vi "Eurotherm_2023_Module.vi"(4 "Decimales":u16(ring)=1 items=["0"=1, "1"=10, "2"=100], 5 "Eurotherm (T:Enable)":bool=TRUE, 6 "delay(s)":dbl=0.15 format="%#_13g", 7 "Command":T3, 8 "error in (no error)":errorcluster, 9 "Value":dbl format="%04.1g", 10 "Address":T1, 11 "VISA resource name":refnum<visa-resource-name>) -> (0 "error out":errorcluster, 2 "Eurotherm":T2, 3 "Valid":bool)   [LabVIEW 2017]
uses:
  Eurotherm_2023_Module.ctl
  Address.ctl
  <vilib>/Instr/_visa.llb/VISA Configure Serial Port (Instr).vi
panel:
  out "String Read":string
  out "String Write":string
  # "NUEVO MODULO VI\nQUE INCORPORA LÍMITES DE SALIDA"
  # "Eurotherm New Module"
  # "Input Data"
  # "Local Data"
  # "Output Data"
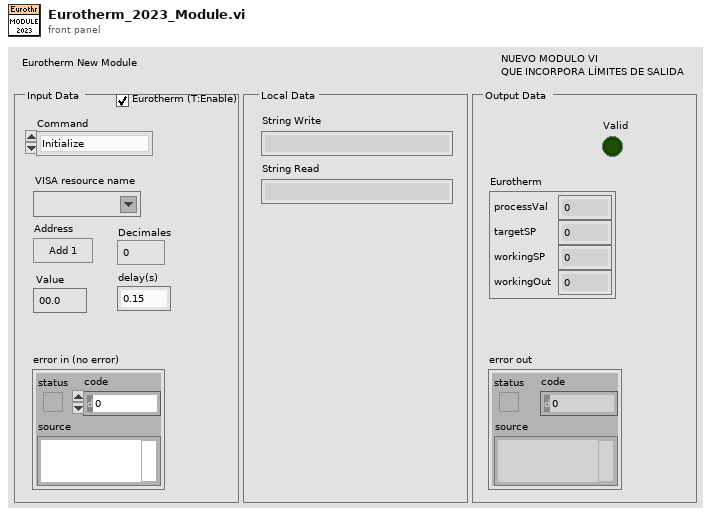
[diagram p1: front panel]
types:
  T1 = typedef "Address.ctl" = enum16{"Add 1", "Add 2", "Add 3", "Add 4", "Add 5", "Add 6", "Add 10", "Add 11", "Add 12", "Add 13"}
  T2 = cluster{"processVal":dbl, "targetSP":dbl, "workingSP":dbl, "workingOut":dbl}
  T3 = typedef "Eurotherm_2023_Module.ctl" = enum16{"Initialize", "Write setpoint", "Read data", "Write ramp rate", "Set constante proporcional", "Set constante integral", "Set constante diferencial", "Set ouput limit LOW", "Set ouput limit HIGH", "Shutdown"}
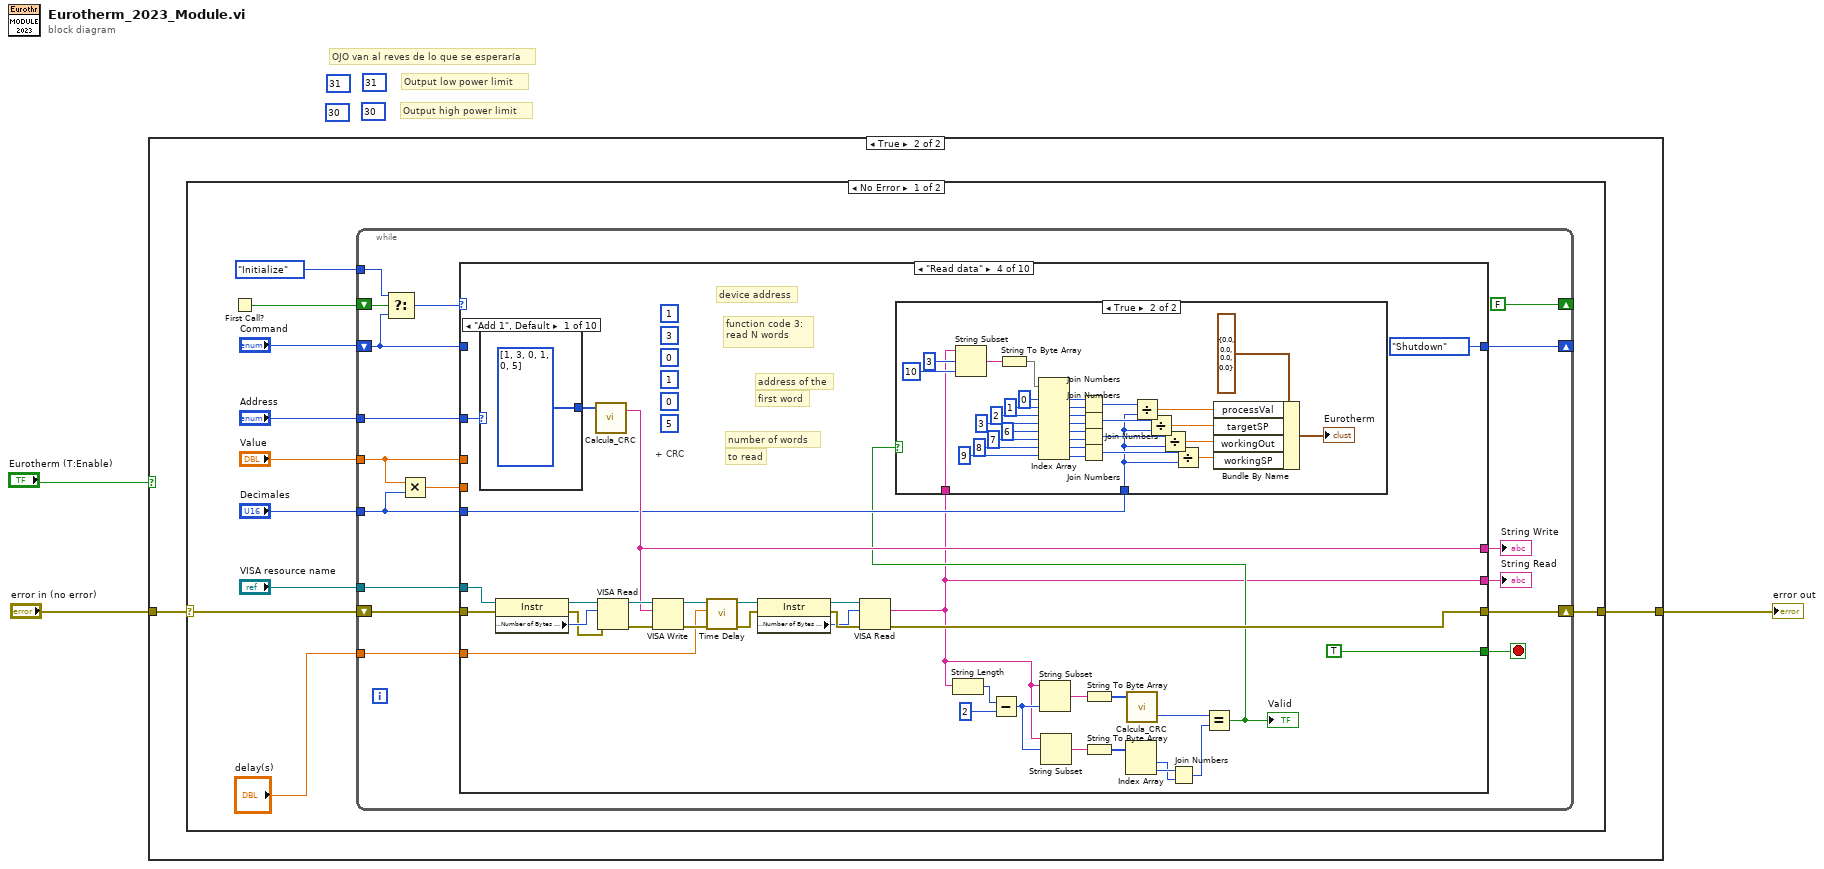
[diagram p0: block diagram]
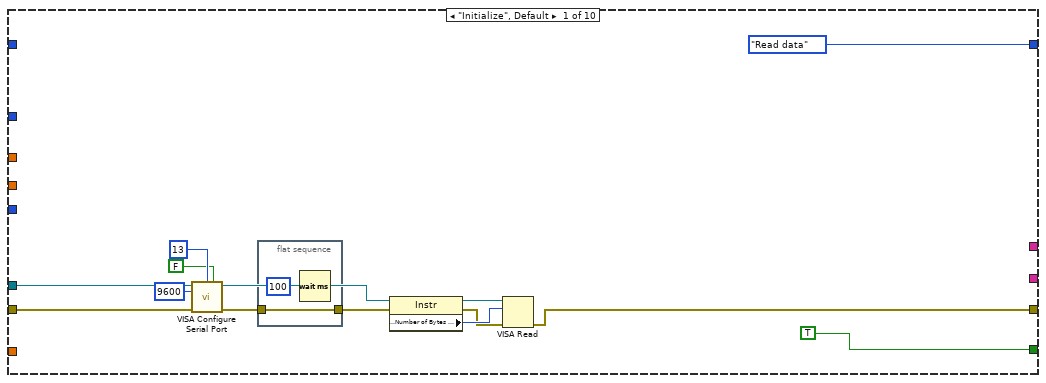
[diagram p3: hidden frame]
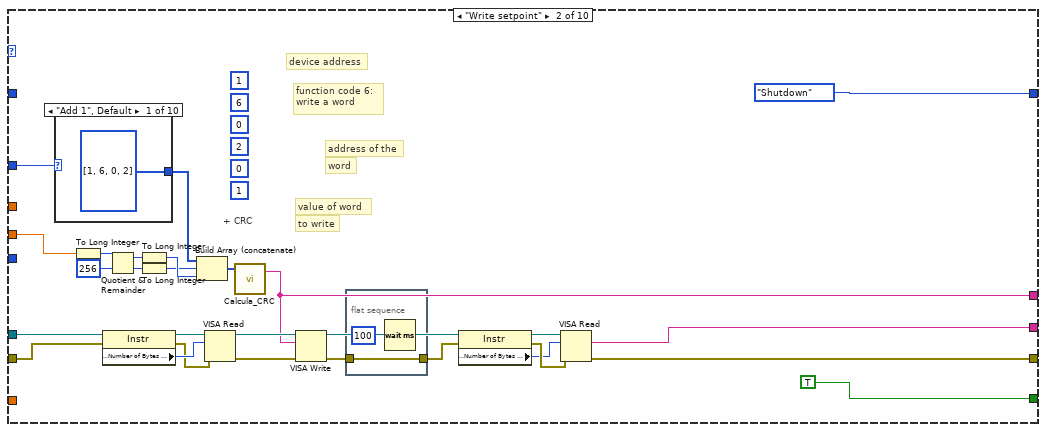
[diagram p4: hidden frame]
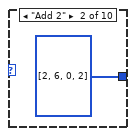
[diagram p5: hidden frame]
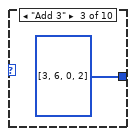
[diagram p6: hidden frame]
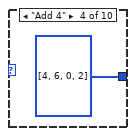
[diagram p7: hidden frame]
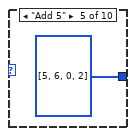
[diagram p8: hidden frame]
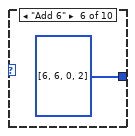
[diagram p9: hidden frame]
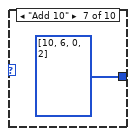
[diagram p10: hidden frame]
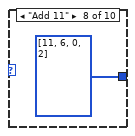
[diagram p11: hidden frame]
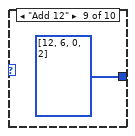
[diagram p12: hidden frame]
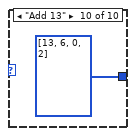
[diagram p13: hidden frame]
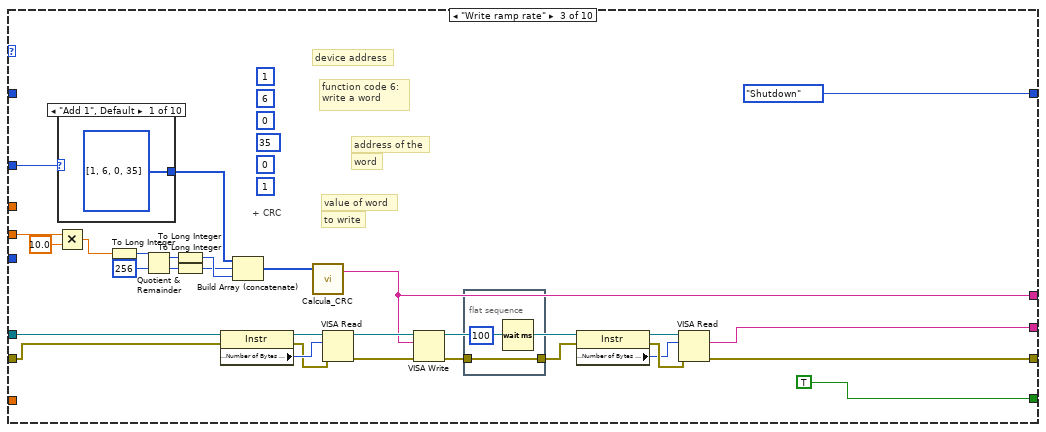
[diagram p14: hidden frame]
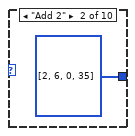
[diagram p15: hidden frame]
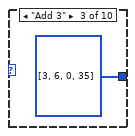
[diagram p16: hidden frame]
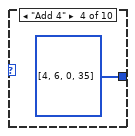
[diagram p17: hidden frame]
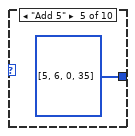
[diagram p18: hidden frame]
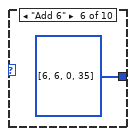
[diagram p19: hidden frame]
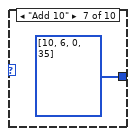
[diagram p20: hidden frame]
diagram:
  (unwired) u8 30
  (unwired) u8 31
  (unwired) u8 30
  (unwired) u8 31
  # "OJO van al reves de lo que se esperaría"
  # "Output high power limit"
  # "Output low power limit"
  n1 = case shown="True" "Eurotherm (T:Enable)" {
    tunnel: "error in (no error)" -> [w4 w6]
    tunnel: [w4 w5] -> w2
    frame False {
    }
    frame True {
      n2 = case shown="No Error" w6 {
        selector: w6 -> [w15 w413]
        tunnel: [w14 w413] -> w5
        frame No Error {
          n3 = First Call?() -> (First Call?: T/F=w16:bool)
          n4 = while {
            shift-right: [w28] -> _
            shift-left: "Command" -> [w29]
            shift-right: [w26] -> w14
            shift-left: w15 -> [w25]
            shift-right: [FALSE ("First Call?: T/F")] -> _
            shift-left: w16 -> [w33]
            tunnel: Eurotherm_2023_Module."Initialize" ("Command") -> [w32]
            tunnel: "Address" -> [w22]
            tunnel: "Value" -> [w19]
            tunnel: "Decimales" -> [w21]
            tunnel: "VISA resource name" -> [w18]
            tunnel: "delay(s)" -> [w17]
            stop <- w27 stop-if-true
            n5 = Select(t=w32, s=w33, f=w29) -> (s? t:f=w30:T3)
            n6 = Multiply(x=w19, y=w21) -> (x*y=w20:dbl)
            n7 = case shown="\"Read data\"" w30 {
              tunnel: w29 -> [_ _ _ _ _ _ _ _ _ _]
              tunnel: [Eurotherm_2023_Module."Read data" ("Command") Eurotherm_2023_Module."Shutdown" ("Command") Eurotherm_2023_Module."Shutdown" ("Command") Eurotherm_2023_Module."Shutdown" ("Command") Eurotherm_2023_Module."Shutdown" ("Command") Eurotherm_2023_Module."Shutdown" ("Command") Eurotherm_2023_Module."Shutdown" ("Command") Eurotherm_2023_Module."Shutdown" ("Command") Eurotherm_2023_Module."Shutdown" ("Command") Eurotherm_2023_Module."Shutdown" ("Command")] -> w28
              tunnel: [TRUE ("First Call?: T/F") TRUE ("First Call?: T/F") TRUE ("First Call?: T/F") TRUE ("First Call?: T/F") TRUE ("First Call?: T/F") TRUE ("First Call?: T/F") TRUE ("First Call?: T/F") TRUE ("First Call?: T/F") TRUE ("First Call?: T/F") TRUE ("First Call?: T/F")] -> w27
              tunnel: [w37 w57 w96 w150 w215 w255 w295 w335 w375 w409] -> w26
              tunnel: w25 -> [w38 w58 w99 w154 w216 w256 w296 w336 w376 w410]
              tunnel: w18 -> [w35 w56 w100 w153 w214 w254 w294 w334 w374 w411]
              tunnel: [_ w55 w95 w132 w213 w253 w293 w333 w373 _] -> w24
              tunnel: [_ w54 w94 w152 w212 w252 w292 w332 w372 _] -> w23
              tunnel: w22 -> [_ w52 w98 w165 w210 w250 w290 w330 w370 _]
              tunnel: w20 -> [_ w51 w93 _ _ _ _ _ _ _]
              tunnel: w21 -> [_ _ _ w146 _ _ _ _ _ _]
              tunnel: w19 -> [_ _ _ _ w209 w249 w289 w329 w369 _]
              tunnel: w17 -> [_ _ _ w147 _ _ _ _ _ _]
              frame "Initialize", Default {
                n8 = call-poly "VISA Configure Serial Port"("VISA resource name"=w35, "termination char\n(0xA = '\\n' = LF)"=u8 13 ("termination char\n(0xA = '\\n' = LF)"), "Enable Termination\nChar (T)"=FALSE ("Enable Termination\nChar (T)"), "baud rate (9600)"=u32 9600, "error in (no error)"=w38) -> ("VISA resource name out"=w39:refnum<visa-resource-name>, "error out"=w40:errorcluster)  [unwired: 9 in]
                n9 = flat-sequence {
                  tunnel: w40 -> [w48]
                  tunnel: [w48] -> w47
                  frame #0 {
                    n10 = Wait (ms)(milliseconds to wait=u32 100) -> ()  [unwired: 1 out]
                  }
                }
                n11 = property class="Instr"(reference=w39, error in=w47) -> (reference out=w44:refnum<visa-resource-name>, error out=w45:errorcluster, "Serial Settings:Number of Bytes at Serial Port"=w46:u32)
                n12 = VISA Read(VISA resource name=w44, byte count=w46, error in (no error)=w45) -> (error out=w37:errorcluster)  [unwired: 3 out]
              }
              frame "Write setpoint" {
                (unwired) 1
                (unwired) u8 0
                (unwired) 2
                (unwired) u8 0
                (unwired) 6
                (unwired) u8 1
                # "+ CRC"
                # "to write"
                # "value of word"
                # "word"
                # "address of the"
                # "function code 6:\nwrite a word"
                # "device address"
                n13 = case shown="\"Add 1\", Default" w52 {
                  tunnel: [u8[] [1, 6, 0, 2] ("Message Data") u8[] [2, 6, 0, 2] ("Message Data") u8[] [3, 6, 0, 2] ("Message Data") u8[] [4, 6, 0, 2] ("Message Data") u8[] [5, 6, 0, 2] ("Message Data") u8[] [6, 6, 0, 2] ("Message Data") u8[] [10, 6, 0, 2] ("Message Data") u8[] [11, 6, 0, 2] ("Message Data") u8[] [12, 6, 0, 2] ("Message Data") u8[] [13, 6, 0, 2] ("Message Data")] -> w77
                  frame "Add 1", Default {
                  }
                  frame "Add 2" {
                  }
                  frame "Add 3" {
                  }
                  frame "Add 4" {
                  }
                  frame "Add 5" {
                  }
                  frame "Add 6" {
                  }
                  frame "Add 10" {
                  }
                  frame "Add 11" {
                  }
                  frame "Add 12" {
                  }
                  frame "Add 13" {
                  }
                }
                n14 = To Long Integer(number=w51) -> (32bit integer=w76:i32)
                n15 = property class="Instr"(reference=w56, error in=w58) -> (reference out=w59:refnum<visa-resource-name>, error out=w60:errorcluster, "Serial Settings:Number of Bytes at Serial Port"=w61:u32)
                n16 = Quotient & Remainder(x=w76, y=256) -> (x-y*floor(x/y)=w71:i32, floor(x/y)=w72:i32)
                n17 = To Long Integer(number=w71) -> (32bit integer=w74:i32)
                n18 = To Long Integer(number=w72) -> (32bit integer=w73:i32)
                n19 = Build Array (concatenate)(w77, w73, w74) -> (w75:i32[])
                n20 = VISA Read(VISA resource name=w59, byte count=w61, error in (no error)=w60) -> (VISA resource name out=w68:refnum<visa-resource-name>, error out=w67:errorcluster)  [unwired: 2 out]
                n21 = call "Calcula_CRC.vi"("Message Data"=w75) -> ("String"=w54:string)  [unwired: 2 in, 1 out]
                n22 = VISA Write(VISA resource name=w68, write buffer=w54, error in (no error)=w67) -> (VISA resource name out=w69:refnum<visa-resource-name>, error out=w66:errorcluster)  [unwired: 1 out]
                n23 = flat-sequence {
                  tunnel: w66 -> [w78]
                  tunnel: [w78] -> w65
                  frame #0 {
                    n24 = Wait (ms)(milliseconds to wait=u32 100) -> ()  [unwired: 1 out]
                  }
                }
                n25 = property class="Instr"(reference=w69, error in=w65) -> (reference out=w64:refnum<visa-resource-name>, error out=w63:errorcluster, "Serial Settings:Number of Bytes at Serial Port"=w62:u32)
                n26 = VISA Read(VISA resource name=w64, byte count=w62, error in (no error)=w63) -> (read buffer=w55:string, error out=w57:errorcluster)  [unwired: 2 out]
              }
              frame "Write ramp rate" {
                (unwired) 1
                (unwired) u8 0
                (unwired) 35
                (unwired) u8 0
                (unwired) 6
                (unwired) u8 1
                # "+ CRC"
                # "to write"
                # "value of word"
                # "word"
                # "address of the"
                # "function code 6:\nwrite a word"
                # "device address"
                n27 = Multiply(x=w93, y=10.0) -> (x*y=w92:dbl)
                n28 = case shown="\"Add 1\", Default" w98 {
                  tunnel: [u8[] [1, 6, 0, 35] ("Message Data") u8[] [2, 6, 0, 35] ("Message Data") u8[] [3, 6, 0, 35] ("Message Data") u8[] [4, 6, 0, 35] ("Message Data") u8[] [5, 6, 0, 35] ("Message Data") u8[] [6, 6, 0, 35] ("Message Data") u8[] [10, 6, 0, 35] ("Message Data") u8[] [11, 6, 0, 35] ("Message Data") u8[] [12, 6, 0, 35] ("Message Data") u8[] [13, 6, 0, 35] ("Message Data")] -> w119
                  frame "Add 1", Default {
                  }
                  frame "Add 2" {
                  }
                  frame "Add 3" {
                  }
                  frame "Add 4" {
                  }
                  frame "Add 5" {
                  }
                  frame "Add 6" {
                  }
                  frame "Add 10" {
                  }
                  frame "Add 11" {
                  }
                  frame "Add 12" {
                  }
                  frame "Add 13" {
                  }
                }
                n29 = To Long Integer(number=w92) -> (32bit integer=w118:i32)
                n30 = Quotient & Remainder(x=w118, y=256) -> (x-y*floor(x/y)=w113:i32, floor(x/y)=w114:i32)
                n31 = To Long Integer(number=w113) -> (32bit integer=w116:i32)
                n32 = To Long Integer(number=w114) -> (32bit integer=w115:i32)
                n33 = property class="Instr"(reference=w100, error in=w99) -> (reference out=w101:refnum<visa-resource-name>, error out=w102:errorcluster, "Serial Settings:Number of Bytes at Serial Port"=w103:u32)
                n34 = Build Array (concatenate)(w119, w115, w116) -> (w117:i32[])
                n35 = call "Calcula_CRC.vi"("Message Data"=w117) -> ("String"=w94:string)  [unwired: 2 in, 1 out]
                n36 = VISA Read(VISA resource name=w101, byte count=w103, error in (no error)=w102) -> (VISA resource name out=w110:refnum<visa-resource-name>, error out=w109:errorcluster)  [unwired: 2 out]
                n37 = VISA Write(VISA resource name=w110, write buffer=w94, error in (no error)=w109) -> (VISA resource name out=w111:refnum<visa-resource-name>, error out=w108:errorcluster)  [unwired: 1 out]
                n38 = flat-sequence {
                  tunnel: w108 -> [w120]
                  tunnel: [w120] -> w107
                  frame #0 {
                    n39 = Wait (ms)(milliseconds to wait=u32 100) -> ()  [unwired: 1 out]
                  }
                }
                n40 = property class="Instr"(reference=w111, error in=w107) -> (reference out=w106:refnum<visa-resource-name>, error out=w105:errorcluster, "Serial Settings:Number of Bytes at Serial Port"=w104:u32)
                n41 = VISA Read(VISA resource name=w106, byte count=w104, error in (no error)=w105) -> (read buffer=w95:string, error out=w96:errorcluster)  [unwired: 2 out]
              }
              frame "Read data" {
                (unwired) u8 5
                (unwired) u8 0
                (unwired) u8 1
                (unwired) u8 0
                (unwired) u8 3
                (unwired) u8 1
                # "+ CRC"
                # "to read"
                # "number of words"
                # "first word"
                # "address of the"
                # "function code 3:\nread N words"
                # "device address"
                n42 = case shown="\"Add 1\", Default" w165 {
                  tunnel: [u8[] [1, 3, 0, 1, 0, 5] ("Message Data") u8[] [2, 3, 0, 1, 0, 5] ("Message Data") u8[] [3, 3, 0, 1, 0, 5] ("Message Data") u8[] [4, 3, 0, 1, 0, 5] ("Message Data") u8[] [5, 3, 0, 1, 0, 5] ("Message Data") u8[] [6, 3, 0, 1, 0, 5] ("Message Data") u8[] [10, 3, 0, 1, 0, 5] ("Message Data") u8[] [11, 3, 0, 1, 0, 5] ("Message Data") u8[] [12, 3, 0, 1, 0, 5] ("Message Data") u8[] [13, 3, 0, 1, 0, 5] ("Message Data")] -> w164
                  frame "Add 1", Default {
                  }
                  frame "Add 2" {
                  }
                  frame "Add 3" {
                  }
                  frame "Add 4" {
                  }
                  frame "Add 5" {
                  }
                  frame "Add 6" {
                  }
                  frame "Add 10" {
                  }
                  frame "Add 11" {
                  }
                  frame "Add 12" {
                  }
                  frame "Add 13" {
                  }
                }
                n43 = property class="Instr"(reference=w153, error in=w154) -> (reference out=w155:refnum<visa-resource-name>, error out=w156:errorcluster, "Serial Settings:Number of Bytes at Serial Port"=w157:u32)
                n44 = call "Calcula_CRC.vi"("Message Data"=w164) -> ("String"=w152:string)  [unwired: 2 in, 1 out]
                n45 = VISA Read(VISA resource name=w155, byte count=w157, error in (no error)=w156) -> (VISA resource name out=w162:refnum<visa-resource-name>, error out=w161:errorcluster)  [unwired: 2 out]
                n46 = VISA Write(VISA resource name=w162, write buffer=w152, error in (no error)=w161) -> (VISA resource name out=w163:refnum<visa-resource-name>, error out=w149:errorcluster)  [unwired: 1 out]
                n47 = call "Time Delay"("error in (no error)"=w149, "Delay Time (s)"=w147) -> ("error out"=w148:errorcluster)  [unwired: 9 in]
                n48 = property class="Instr"(reference=w163, error in=w148) -> (reference out=w160:refnum<visa-resource-name>, error out=w159:errorcluster, "Serial Settings:Number of Bytes at Serial Port"=w158:u32)
                n49 = VISA Read(VISA resource name=w160, byte count=w158, error in (no error)=w159) -> (read buffer=w132:string, error out=w150:errorcluster)  [unwired: 2 out]
                n50 = String Length(string=w132) -> (length=w144:i32)
                n51 = Subtract(x=w144, y=2) -> (x-y=w143:i32)
                n52 = String Subset(string=w132, length (rest)=w143) -> (substring=w142:string)  [unwired: 1 in]
                n53 = String Subset(string=w132, offset (0)=w143) -> (substring=w140:string)  [unwired: 1 in]
                n54 = String To Byte Array(string=w142) -> (unsigned byte array=w141:u8[])
                n55 = String To Byte Array(string=w140) -> (unsigned byte array=w139:u8[])
                n56 = Index Array(array=w139) -> (element #1=w137:u8, element #2=w138:u8)  [unwired: 2 in]
                n57 = call "Calcula_CRC.vi"("Message Data"=w141) -> ("Calculated CRC"=w136:u16)  [unwired: 2 in, 1 out]
                n58 = Join Numbers(hi=w138, lo=w137) -> ((hi.lo)=w135:u16)
                n59 = Equal?(x=w136, y=w135) -> (x = y?=w133:bool)
                "Valid" <- w133
                n60 = case shown="True" w133 {
                  tunnel: w132 -> [_ w191]
                  tunnel: w146 -> [_ w172]
                  frame False {
                  }
                  frame True {
                    n61 = String Subset(string=w191, offset (0)=3, length (rest)=10 ("length (rest)")) -> (substring=w192:string)
                    n62 = String To Byte Array(string=w192) -> (unsigned byte array=w195:u8[])
                    n63 = Index Array(array=w195, index #1=0 ("index"), index #2=1 ("index"), index #3=2 ("index"), index #4=3 ("index"), index #5=6 ("index"), index #6=7 ("index"), index #7=8 ("index"), index #8=9 ("index")) -> (element #1=w184:u8, element #2=w183:u8, element #3=w182:u8, element #4=w181:u8, element #5=w180:u8, element #6=w179:u8, element #7=w178:u8, element #8=w177:u8)
                    n64 = Join Numbers(hi=w184, lo=w183) -> ((hi.lo)=w176:u16)
                    n65 = Join Numbers(hi=w182, lo=w181) -> ((hi.lo)=w175:u16)
                    n66 = Join Numbers(hi=w180, lo=w179) -> ((hi.lo)=w174:u16)
                    n67 = Join Numbers(hi=w178, lo=w177) -> ((hi.lo)=w173:u16)
                    n68 = Divide(x=w176, y=w172) -> (x/y=w166:dbl)
                    n69 = Divide(x=w175, y=w172) -> (x/y=w167:dbl)
                    n70 = Divide(x=w174, y=w172) -> (x/y=w168:dbl)
                    n71 = Divide(x=w173, y=w172) -> (x/y=w169:dbl)
                    n72 = Bundle By Name(cluster=T2 {"processVal"=0.0, "targetSP"=0.0, "workingSP"=0.0, "workingOut"=0.0} ("Eurotherm"), "processVal"=w166, "targetSP"=w167, "workingOut"=w168, "workingSP"=w169) -> (→"Eurotherm":T2)
                  }
                }
              }
              frame "Set constante proporcional" {
                (unwired) 1
                (unwired) u8 0
                (unwired) 6
                (unwired) u8 0
                (unwired) 6
                (unwired) u8 1
                # "+ CRC"
                # "to write"
                # "value of word"
                # "word"
                # "address of the"
                # "function code 6:\nwrite a word"
                # "device address"
                n73 = case shown="\"Add 1\", Default" w210 {
                  tunnel: [u8[] [1, 6, 0, 6] ("Message Data") u8[] [2, 6, 0, 6] ("Message Data") u8[] [3, 6, 0, 6] ("Message Data") u8[] [4, 6, 0, 6] ("Message Data") u8[] [5, 6, 0, 6] ("Message Data") u8[] [6, 6, 0, 6] ("Message Data") u8[] [10, 6, 0, 6] ("Message Data") u8[] [11, 6, 0, 6] ("Message Data") u8[] [12, 6, 0, 6] ("Message Data") u8[] [13, 6, 0, 6] ("Message Data")] -> w235
                  frame "Add 1", Default {
                  }
                  frame "Add 2" {
                  }
                  frame "Add 3" {
                  }
                  frame "Add 4" {
                  }
                  frame "Add 5" {
                  }
                  frame "Add 6" {
                  }
                  frame "Add 10" {
                  }
                  frame "Add 11" {
                  }
                  frame "Add 12" {
                  }
                  frame "Add 13" {
                  }
                }
                n74 = To Long Integer(number=w209) -> (32bit integer=w234:i32)
                n75 = property class="Instr"(reference=w214, error in=w216) -> (reference out=w217:refnum<visa-resource-name>, error out=w218:errorcluster, "Serial Settings:Number of Bytes at Serial Port"=w219:u32)
                n76 = Quotient & Remainder(x=w234, y=256) -> (x-y*floor(x/y)=w229:i32, floor(x/y)=w230:i32)
                n77 = To Long Integer(number=w229) -> (32bit integer=w232:i32)
                n78 = To Long Integer(number=w230) -> (32bit integer=w231:i32)
                n79 = Build Array (concatenate)(w235, w231, w232) -> (w233:i32[])
                n80 = VISA Read(VISA resource name=w217, byte count=w219, error in (no error)=w218) -> (VISA resource name out=w226:refnum<visa-resource-name>, error out=w225:errorcluster)  [unwired: 2 out]
                n81 = call "Calcula_CRC.vi"("Message Data"=w233) -> ("String"=w212:string)  [unwired: 2 in, 1 out]
                n82 = VISA Write(VISA resource name=w226, write buffer=w212, error in (no error)=w225) -> (VISA resource name out=w227:refnum<visa-resource-name>, error out=w224:errorcluster)  [unwired: 1 out]
                n83 = flat-sequence {
                  tunnel: w224 -> [w236]
                  tunnel: [w236] -> w223
                  frame #0 {
                    n84 = Wait (ms)(milliseconds to wait=u32 100) -> ()  [unwired: 1 out]
                  }
                }
                n85 = property class="Instr"(reference=w227, error in=w223) -> (reference out=w222:refnum<visa-resource-name>, error out=w221:errorcluster, "Serial Settings:Number of Bytes at Serial Port"=w220:u32)
                n86 = VISA Read(VISA resource name=w222, byte count=w220, error in (no error)=w221) -> (read buffer=w213:string, error out=w215:errorcluster)  [unwired: 2 out]
              }
              frame "Set constante integral" {
                (unwired) 1
                (unwired) u8 0
                (unwired) 8
                (unwired) u8 0
                (unwired) 6
                (unwired) u8 1
                # "+ CRC"
                # "to write"
                # "value of word"
                # "word"
                # "address of the"
                # "function code 6:\nwrite a word"
                # "device address"
                n87 = case shown="\"Add 1\", Default" w250 {
                  tunnel: [u8[] [1, 6, 0, 8] ("Message Data") u8[] [2, 6, 0, 8] ("Message Data") u8[] [3, 6, 0, 8] ("Message Data") u8[] [4, 6, 0, 8] ("Message Data") u8[] [5, 6, 0, 8] ("Message Data") u8[] [6, 6, 0, 8] ("Message Data") u8[] [10, 6, 0, 8] ("Message Data") u8[] [11, 6, 0, 8] ("Message Data") u8[] [12, 6, 0, 8] ("Message Data") u8[] [13, 6, 0, 8] ("Message Data")] -> w275
                  frame "Add 1", Default {
                  }
                  frame "Add 2" {
                  }
                  frame "Add 3" {
                  }
                  frame "Add 4" {
                  }
                  frame "Add 5" {
                  }
                  frame "Add 6" {
                  }
                  frame "Add 10" {
                  }
                  frame "Add 11" {
                  }
                  frame "Add 12" {
                  }
                  frame "Add 13" {
                  }
                }
                n88 = To Long Integer(number=w249) -> (32bit integer=w274:i32)
                n89 = property class="Instr"(reference=w254, error in=w256) -> (reference out=w257:refnum<visa-resource-name>, error out=w258:errorcluster, "Serial Settings:Number of Bytes at Serial Port"=w259:u32)
                n90 = Quotient & Remainder(x=w274, y=256) -> (x-y*floor(x/y)=w269:i32, floor(x/y)=w270:i32)
                n91 = To Long Integer(number=w269) -> (32bit integer=w272:i32)
                n92 = To Long Integer(number=w270) -> (32bit integer=w271:i32)
                n93 = Build Array (concatenate)(w275, w271, w272) -> (w273:i32[])
                n94 = VISA Read(VISA resource name=w257, byte count=w259, error in (no error)=w258) -> (VISA resource name out=w266:refnum<visa-resource-name>, error out=w265:errorcluster)  [unwired: 2 out]
                n95 = call "Calcula_CRC.vi"("Message Data"=w273) -> ("String"=w252:string)  [unwired: 2 in, 1 out]
                n96 = VISA Write(VISA resource name=w266, write buffer=w252, error in (no error)=w265) -> (VISA resource name out=w267:refnum<visa-resource-name>, error out=w264:errorcluster)  [unwired: 1 out]
                n97 = flat-sequence {
                  tunnel: w264 -> [w276]
                  tunnel: [w276] -> w263
                  frame #0 {
                    n98 = Wait (ms)(milliseconds to wait=u32 100) -> ()  [unwired: 1 out]
                  }
                }
                n99 = property class="Instr"(reference=w267, error in=w263) -> (reference out=w262:refnum<visa-resource-name>, error out=w261:errorcluster, "Serial Settings:Number of Bytes at Serial Port"=w260:u32)
                n100 = VISA Read(VISA resource name=w262, byte count=w260, error in (no error)=w261) -> (read buffer=w253:string, error out=w255:errorcluster)  [unwired: 2 out]
              }
              frame "Set constante diferencial" {
                (unwired) 1
                (unwired) u8 0
                (unwired) 9
                (unwired) u8 0
                (unwired) 6
                (unwired) u8 1
                # "+ CRC"
                # "to write"
                # "value of word"
                # "word"
                # "address of the"
                # "function code 6:\nwrite a word"
                # "device address"
                n101 = case shown="\"Add 1\", Default" w290 {
                  tunnel: [u8[] [1, 6, 0, 9] ("Message Data") u8[] [2, 6, 0, 9] ("Message Data") u8[] [3, 6, 0, 9] ("Message Data") u8[] [4, 6, 0, 9] ("Message Data") u8[] [5, 6, 0, 9] ("Message Data") u8[] [6, 6, 0, 9] ("Message Data") u8[] [10, 6, 0, 9] ("Message Data") u8[] [11, 6, 0, 9] ("Message Data") u8[] [12, 6, 0, 9] ("Message Data") u8[] [13, 6, 0, 9] ("Message Data")] -> w315
                  frame "Add 1", Default {
                  }
                  frame "Add 2" {
                  }
                  frame "Add 3" {
                  }
                  frame "Add 4" {
                  }
                  frame "Add 5" {
                  }
                  frame "Add 6" {
                  }
                  frame "Add 10" {
                  }
                  frame "Add 11" {
                  }
                  frame "Add 12" {
                  }
                  frame "Add 13" {
                  }
                }
                n102 = To Long Integer(number=w289) -> (32bit integer=w314:i32)
                n103 = property class="Instr"(reference=w294, error in=w296) -> (reference out=w297:refnum<visa-resource-name>, error out=w298:errorcluster, "Serial Settings:Number of Bytes at Serial Port"=w299:u32)
                n104 = Quotient & Remainder(x=w314, y=256) -> (x-y*floor(x/y)=w309:i32, floor(x/y)=w310:i32)
                n105 = To Long Integer(number=w309) -> (32bit integer=w312:i32)
                n106 = To Long Integer(number=w310) -> (32bit integer=w311:i32)
                n107 = Build Array (concatenate)(w315, w311, w312) -> (w313:i32[])
                n108 = VISA Read(VISA resource name=w297, byte count=w299, error in (no error)=w298) -> (VISA resource name out=w306:refnum<visa-resource-name>, error out=w305:errorcluster)  [unwired: 2 out]
                n109 = call "Calcula_CRC.vi"("Message Data"=w313) -> ("String"=w292:string)  [unwired: 2 in, 1 out]
                n110 = VISA Write(VISA resource name=w306, write buffer=w292, error in (no error)=w305) -> (VISA resource name out=w307:refnum<visa-resource-name>, error out=w304:errorcluster)  [unwired: 1 out]
                n111 = flat-sequence {
                  tunnel: w304 -> [w316]
                  tunnel: [w316] -> w303
                  frame #0 {
                    n112 = Wait (ms)(milliseconds to wait=u32 100) -> ()  [unwired: 1 out]
                  }
                }
                n113 = property class="Instr"(reference=w307, error in=w303) -> (reference out=w302:refnum<visa-resource-name>, error out=w301:errorcluster, "Serial Settings:Number of Bytes at Serial Port"=w300:u32)
                n114 = VISA Read(VISA resource name=w302, byte count=w300, error in (no error)=w301) -> (read buffer=w293:string, error out=w295:errorcluster)  [unwired: 2 out]
              }
              frame "Set ouput limit LOW" {
                (unwired) 1
                (unwired) u8 0
                (unwired) 31
                (unwired) u8 0
                (unwired) 6
                (unwired) u8 1
                # "+ CRC"
                # "to write"
                # "value of word"
                # "word"
                # "address of the"
                # "function code 6:\nwrite a word"
                # "device address"
                n115 = case shown="\"Add 1\", Default" w330 {
                  tunnel: [u8[] [1, 6, 0, 31] ("Message Data") u8[] [2, 6, 0, 31] ("Message Data") u8[] [3, 6, 0, 31] ("Message Data") u8[] [4, 6, 0, 31] ("Message Data") u8[] [5, 6, 0, 31] ("Message Data") u8[] [6, 6, 0, 31] ("Message Data") u8[] [10, 6, 0, 31] ("Message Data") u8[] [11, 6, 0, 31] ("Message Data") u8[] [12, 6, 0, 31] ("Message Data") u8[] [13, 6, 0, 31] ("Message Data")] -> w355
                  frame "Add 1", Default {
                  }
                  frame "Add 2" {
                  }
                  frame "Add 3" {
                  }
                  frame "Add 4" {
                  }
                  frame "Add 5" {
                  }
                  frame "Add 6" {
                  }
                  frame "Add 10" {
                  }
                  frame "Add 11" {
                  }
                  frame "Add 12" {
                  }
                  frame "Add 13" {
                  }
                }
                n116 = To Long Integer(number=w329) -> (32bit integer=w354:i32)
                n117 = property class="Instr"(reference=w334, error in=w336) -> (reference out=w337:refnum<visa-resource-name>, error out=w338:errorcluster, "Serial Settings:Number of Bytes at Serial Port"=w339:u32)
                n118 = Quotient & Remainder(x=w354, y=256) -> (x-y*floor(x/y)=w349:i32, floor(x/y)=w350:i32)
                n119 = To Long Integer(number=w349) -> (32bit integer=w352:i32)
                n120 = To Long Integer(number=w350) -> (32bit integer=w351:i32)
                n121 = Build Array (concatenate)(w355, w351, w352) -> (w353:i32[])
                n122 = VISA Read(VISA resource name=w337, byte count=w339, error in (no error)=w338) -> (VISA resource name out=w346:refnum<visa-resource-name>, error out=w345:errorcluster)  [unwired: 2 out]
                n123 = call "Calcula_CRC.vi"("Message Data"=w353) -> ("String"=w332:string)  [unwired: 2 in, 1 out]
                n124 = VISA Write(VISA resource name=w346, write buffer=w332, error in (no error)=w345) -> (VISA resource name out=w347:refnum<visa-resource-name>, error out=w344:errorcluster)  [unwired: 1 out]
                n125 = flat-sequence {
                  tunnel: w344 -> [w356]
                  tunnel: [w356] -> w343
                  frame #0 {
                    n126 = Wait (ms)(milliseconds to wait=u32 100) -> ()  [unwired: 1 out]
                  }
                }
                n127 = property class="Instr"(reference=w347, error in=w343) -> (reference out=w342:refnum<visa-resource-name>, error out=w341:errorcluster, "Serial Settings:Number of Bytes at Serial Port"=w340:u32)
                n128 = VISA Read(VISA resource name=w342, byte count=w340, error in (no error)=w341) -> (read buffer=w333:string, error out=w335:errorcluster)  [unwired: 2 out]
              }
              frame "Set ouput limit HIGH" {
                (unwired) 1
                (unwired) u8 0
                (unwired) 30
                (unwired) u8 0
                (unwired) 6
                (unwired) u8 1
                # "+ CRC"
                # "to write"
                # "value of word"
                # "word"
                # "address of the"
                # "function code 6:\nwrite a word"
                # "device address"
                n129 = case shown="\"Add 1\", Default" w370 {
                  tunnel: [u8[] [1, 6, 0, 30] ("Message Data") u8[] [2, 6, 0, 30] ("Message Data") u8[] [3, 6, 0, 30] ("Message Data") u8[] [4, 6, 0, 30] ("Message Data") u8[] [5, 6, 0, 30] ("Message Data") u8[] [6, 6, 0, 30] ("Message Data") u8[] [10, 6, 0, 30] ("Message Data") u8[] [11, 6, 0, 30] ("Message Data") u8[] [12, 6, 0, 30] ("Message Data") u8[] [13, 6, 0, 30] ("Message Data")] -> w395
                  frame "Add 1", Default {
                  }
                  frame "Add 2" {
                  }
                  frame "Add 3" {
                  }
                  frame "Add 4" {
                  }
                  frame "Add 5" {
                  }
                  frame "Add 6" {
                  }
                  frame "Add 10" {
                  }
                  frame "Add 11" {
                  }
                  frame "Add 12" {
                  }
                  frame "Add 13" {
                  }
                }
                n130 = To Long Integer(number=w369) -> (32bit integer=w394:i32)
                n131 = property class="Instr"(reference=w374, error in=w376) -> (reference out=w377:refnum<visa-resource-name>, error out=w378:errorcluster, "Serial Settings:Number of Bytes at Serial Port"=w379:u32)
                n132 = Quotient & Remainder(x=w394, y=256) -> (x-y*floor(x/y)=w389:i32, floor(x/y)=w390:i32)
                n133 = To Long Integer(number=w389) -> (32bit integer=w392:i32)
                n134 = To Long Integer(number=w390) -> (32bit integer=w391:i32)
                n135 = Build Array (concatenate)(w395, w391, w392) -> (w393:i32[])
                n136 = VISA Read(VISA resource name=w377, byte count=w379, error in (no error)=w378) -> (VISA resource name out=w386:refnum<visa-resource-name>, error out=w385:errorcluster)  [unwired: 2 out]
                n137 = call "Calcula_CRC.vi"("Message Data"=w393) -> ("String"=w372:string)  [unwired: 2 in, 1 out]
                n138 = VISA Write(VISA resource name=w386, write buffer=w372, error in (no error)=w385) -> (VISA resource name out=w387:refnum<visa-resource-name>, error out=w384:errorcluster)  [unwired: 1 out]
                n139 = flat-sequence {
                  tunnel: w384 -> [w396]
                  tunnel: [w396] -> w383
                  frame #0 {
                    n140 = Wait (ms)(milliseconds to wait=u32 100) -> ()  [unwired: 1 out]
                  }
                }
                n141 = property class="Instr"(reference=w387, error in=w383) -> (reference out=w382:refnum<visa-resource-name>, error out=w381:errorcluster, "Serial Settings:Number of Bytes at Serial Port"=w380:u32)
                n142 = VISA Read(VISA resource name=w382, byte count=w380, error in (no error)=w381) -> (read buffer=w373:string, error out=w375:errorcluster)  [unwired: 2 out]
              }
              frame "Shutdown" {
                n143 = VISA Close(VISA resource name=w411, error in (no error)=w410) -> (error out=w409:errorcluster)
              }
            }
            "String Read" <- w24
            "String Write" <- w23
          }
        }
        frame Error {
        }
      }
    }
  }
  "error out" <- w2
